vi "Collate Diff Images.vi"(8 "error in (no error)":errorcluster, 11 "Report XML Path":path) -> (0 "error out":errorcluster, 3 "Collated Directories":path[](array[path]))   [LabVIEW 2020, in "Graphical Diff.lvlib"]
uses:
  Graphical Diff.lvlib
  ae0c8e88-ace4-49d4-90c2-2a76c8cf41b7.vi
  <vilib>/Comparison/Equal/Equal Functor/Equal Functor.lvclass
  <vilib>/xml/NI_XML.lvlib
  <resource>/objmgr/DOMUserDefRef.rc
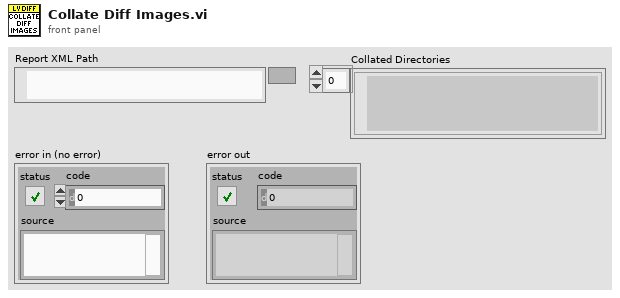
[diagram p1: front panel]
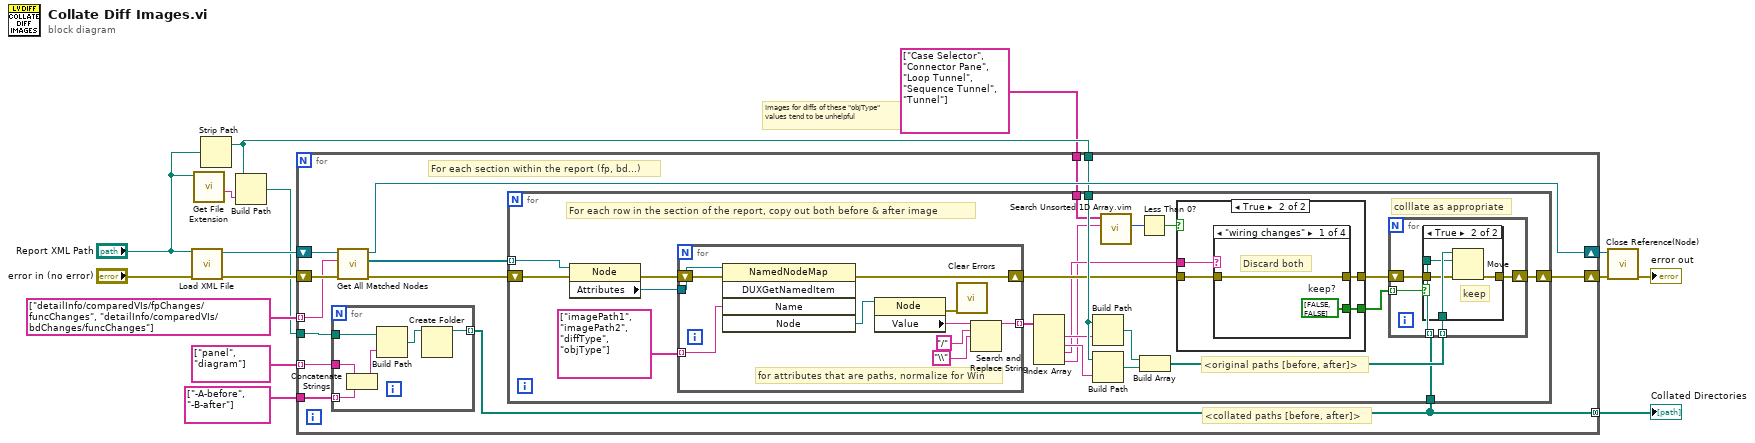
[diagram p0: block diagram]
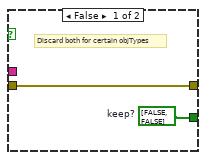
[diagram p2: hidden frame]
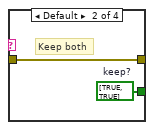
[diagram p3: hidden frame]
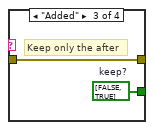
[diagram p4: hidden frame]
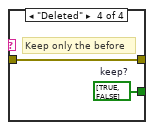
[diagram p5: hidden frame]
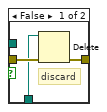
[diagram p6: hidden frame]
diagram:
  # "Images for diffs of these \"objType\" values tend to be unhelpful"
  n1 = call <vilib>:"Load XML File.vi"("path to XML document"="Report XML Path", "error in (no error)"="error in (no error)") -> ("DOM document out"=w15:refnum<k20>, "error out"=w14:errorcluster)  [unwired: 11 in, 1 out]
  n2 = call <vilib>:"Get File Extension.vi"("file"="Report XML Path") -> ("filename without extension"=w11:string)  [unwired: 6 in, 4 out]
  n3 = Strip Path(path="Report XML Path") -> (stripped path=w5:path)  [unwired: 1 out]
  n4 = Build Path(base path=w5, name or relative path=w11) -> (appended path=w4:path)
  n5 = for {
    shift-right: [w21] -> w9
    shift-left: w14 -> [w27]
    shift-right: [w26] -> w10
    shift-left: w15 -> [w28]
    tunnel: string[] ["panel", "diagram"] ("Array 2") -> [w25] mode=indexing
    tunnel: string[] ["detailInfo/comparedVIs/fpChanges/funcChanges", "detailInfo/comparedVIs/bdChanges/funcChanges"] ("Array 2") -> [w24] mode=indexing
    tunnel: w5 -> [w20]
    tunnel: w4 -> [w19]
    tunnel: string[] ["-A-before", "-B-after"] ("Array 2") -> [w18]
    tunnel: [w17] -> w2 mode=concatenating
    tunnel: string[] ["Case Selector", "Connector Pane", "Loop Tunnel", "Sequence Tunnel", "Tunnel"] ("Array 2") -> [w16]
    # "<collated paths [before, after]>"
    # "For each section within the report (fp, bd...)"
    n6 = for {
      tunnel: w25 -> [w89]
      tunnel: w19 -> [w91]
      tunnel: [w90] -> w17 mode=indexing
      tunnel: w18 -> [w88] mode=indexing
      n7 = Concatenate Strings(w89, w88) -> (w87:string)
      n8 = Build Path(base path=w91, name or relative path=w87) -> (appended path=w92:path)
      n9 = Create Folder(path (use dialog)=w92) -> (created path=w90:path)  [unwired: 2 in, 2 out]
    }
    n10 = call <vilib>:"Get All Matched Nodes.vi"("error in (no error)"=w27, "XPath expression"=w24, "node in"=w28) -> ("error out"=w22:errorcluster, "node result array"=w23:refnum<k20>[], "node out"=w26:refnum<k20>)  [unwired: 6 in]
    n11 = for {
      tunnel: w23 -> [w50] mode=indexing
      shift-right: [w36] -> w21
      shift-left: w22 -> [w47]
      tunnel: w17 -> [w33]
      tunnel: w20 -> [w43]
      tunnel: w16 -> [w32]
      # "<original paths [before, after]>"
      # "colllate as appropriate"
      # "For each row in the section of the report, copy out both before & after image"
      n12 = property class="Node"(reference=w50, error in=w47) -> (error out=w48:errorcluster, "Attributes"=w49:refnum<k20>)  [unwired: 1 out]
      n13 = for {
        tunnel: w49 -> [w86]
        tunnel: string[] ["imagePath1", "imagePath2", "diffType", "objType"] ("Array 2") -> [w84] mode=indexing
        shift-right: [w78] -> w40
        shift-left: w48 -> [w85]
        tunnel: [w79] -> w45 mode=indexing
        # "for attributes that are paths, normalize for Win"
        n14 = invoke class="NamedNodeMap" method="DUXGetNamedItem"(reference=w86, error in=w85, "Name"=w84) -> (error out=w78:errorcluster, "Node"=w83:refnum<k20>)  [unwired: 2 in, 3 out]
        n15 = property class="Node"(reference=w83) -> (error out=w77:errorcluster, "Value"=w82:string)  [unwired: 1 in, 1 out]
        n16 = call <vilib>:"Clear Errors.vi"("error in (no error)"=w77) -> ()  [unwired: 5 in, 2 out]
        n17 = Search and Replace String(input string=w82, search string="/", replace string="\\" ("replace string (\"\")")) -> (result string=w79:string)  [unwired: 5 in, 3 out]
      }
      n18 = Index Array(array=w45) -> (element #1=w42:string, element #2=w44:string, element #3=w39:string, element #4=w31:string)  [unwired: 4 in]
      n19 = Build Path(base path=w43, name or relative path=w42) -> (appended path=w38:path)
      n20 = Build Path(base path=w43, name or relative path=w44) -> (appended path=w37:path)
      n21 = call "Search Unsorted 1D Array.vim"("element"=w31, "unsorted 1D array"=w32) -> ("index of element"=w30:i32)  [unwired: 9 in]
      n22 = Less Than 0?(x=w30) -> (x < 0?=w29:bool)
      n23 = Build Array(w38, w37) -> (w35:path[])
      n24 = case shown="True" w29 {
        tunnel: [w52 w56] -> w41
        tunnel: w40 -> [w52 w55]
        tunnel: w39 -> [_ w54]
        tunnel: [w51 w53] -> w34
        frame False {
          w51 = bool[] [FALSE, FALSE]  # keep?
          # "Discard both for certain objTypes"
        }
        frame True {
          n25 = case shown="\"wiring changes\"" w54 {
            tunnel: [w58 w60 w62 w64] -> w56
            tunnel: w55 -> [w58 w60 w62 w64]
            tunnel: [w57 w59 w61 w63] -> w53
            frame "wiring changes" {
              w57 = bool[] [FALSE, FALSE]  # keep?
              # "Discard both"
            }
            frame Default {
              w59 = bool[] [TRUE, TRUE]  # keep?
              # "Keep both"
            }
            frame "Added" {
              w61 = bool[] [FALSE, TRUE]  # keep?
              # "Keep only the after"
            }
            frame "Deleted" {
              w63 = bool[] [TRUE, FALSE]  # keep?
              # "Keep only the before"
            }
          }
        }
      }
      n26 = for {
        shift-right: [w68] -> w36
        shift-left: w41 -> [w69]
        tunnel: w35 -> [w67] mode=indexing
        tunnel: w34 -> [w66] mode=indexing
        tunnel: w33 -> [w65] mode=indexing
        n27 = case shown="True" w66 {
          tunnel: w67 -> [w70 w76]
          tunnel: w69 -> [w72 w75]
          tunnel: [w71 w74] -> w68
          tunnel: w65 -> [_ w73]
          frame False {
            # "discard"
            n28 = Delete(path (use dialog)=w70, error in=w72) -> (error out=w71:errorcluster)  [unwired: 3 in, 2 out]
          }
          frame True {
            # "keep"
            n29 = Move(source path=w76, error in=w75, 10:w73) -> (error out=w74:errorcluster)  [unwired: 2 in, 2 out]
          }
        }
      }
    }
  }
  "Collated Directories" <- w2
  n30 = call <vilib>:"Close Reference(Node).vi"("error in (no error)"=w9, "node"=w10) -> ("error out"=→"error out":errorcluster)  [unwired: 7 in]
